vi "CreateJoystick.vi"(6 "error in (no error)":errorcluster, 8 "refnum name":string="My Joystick RefNum", 9 "JoystickDevice":T1) -> (0 "error out":errorcluster, 3 "JoystickDevRef":T2={"Device"=enum."USB 1"})   [LabVIEW 2014]
uses:
  <vilib>/Rock Robotics/WPI/Joystick/WPI_JoystickDevRef.ctl
  <vilib>/Rock Robotics/WPI/Joystick/WPI_JoystickDeviceEnum.ctl
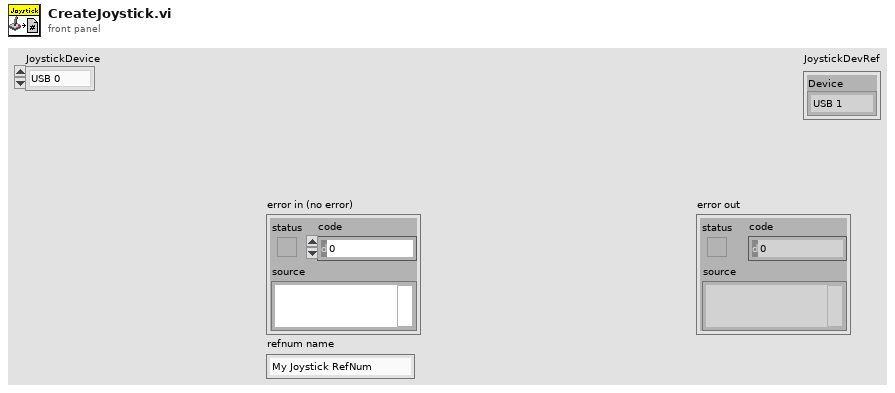
[diagram p1: front panel]
types:
  T1 = typedef "WPI_JoystickDeviceEnum.ctl" = enum16{"USB 0", "USB 1", "USB 2", "USB 3", "USB 4", "USB 5"}
  T2 = typedef "WPI_JoystickDevRef.ctl" = cluster{"Device":T1}
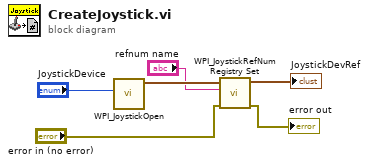
[diagram p0: block diagram]
diagram:
  n1 = call <vilib>:"WPI_JoystickOpen.vi"("JoystickDevice"="JoystickDevice") -> ("JoystickDevRef"=w6:T2)  [unwired: 10 in]
  n2 = call <vilib>:"WPI_JoystickRefNum Registry Set.vi"("error in (no error)"="error in (no error)", "refnum name"="refnum name", "JoystickDevRef"=w6) -> ("error out"=→"error out":errorcluster, "JoystickDevRef"=→"JoystickDevRef":T2)  [unwired: 7 in]
